vi "실습 2-5 난수45.vi"() -> ()   [LabVIEW 2014]
panel:
  out "배열":dbl[](array[numeric])
  out "숫자(0에서 1)":dbl format="%#_15f"
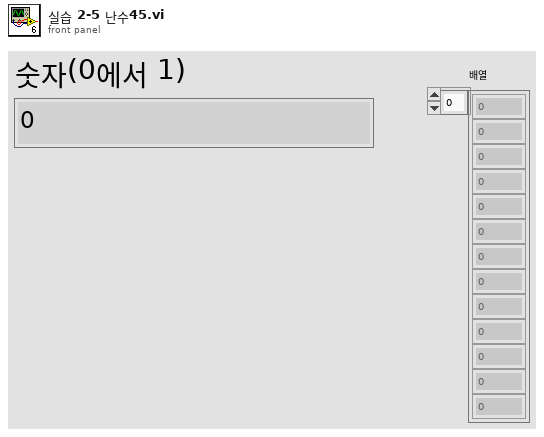
[diagram p1: front panel]
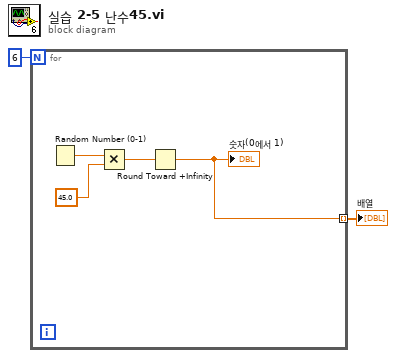
[diagram p0: block diagram]
diagram:
  n1 = for {
    N: 6 -> [_]
    tunnel: [w3] -> w1 mode=indexing
    n2 = Random Number (0-1)() -> (number: 0 to 1=w6:dbl)
    n3 = Multiply(x=w6, y=45.0) -> (x*y=w5:dbl)
    n4 = Round Toward +Infinity(x=w5) -> (ceil(x): smallest int >= x=w3:dbl)
    "숫자(0에서 1)" <- w3
  }
  "배열" <- w1
